vi "readMeasFromFile.vi"(0 "path":path) -> (1 "data":T1(array[cluster]), 2 "Count":i32)   [LabVIEW 2010]
panel:
  out "error out":errorcluster
  in  "MeasData":T2
  in  "Array":string[](array[string])
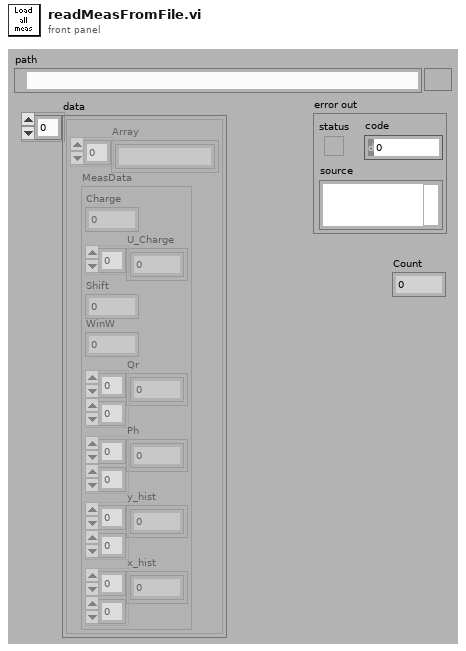
[diagram p1: front panel]
types:
  T1 = cluster{"Array":string[], "MeasData":cluster{"Charge":i32, "U_Charge":i32[], "Shift":i32, "WinW":i32, "Qr":i32[][], "Ph":i32[][], "y_hist":i32[][], "x_hist":i32[][]}}[]
  T2 = cluster{"Charge":i32, "U_Charge":i32[], "Shift":i32, "WinW":i32, "Qr":i32[][], "Ph":i32[][], "y_hist":i32[][], "x_hist":i32[][]}
  T3 = cluster{"Array":string[], "MeasData":cluster{"Charge":i32, "U_Charge":i32[], "Shift":i32, "WinW":i32, "Qr":i32[][], "Ph":i32[][], "y_hist":i32[][], "x_hist":i32[][]}}
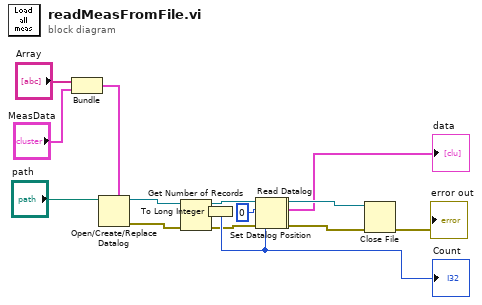
[diagram p0: block diagram]
diagram:
  n1 = Bundle("Array"="Array", "MeasData"="MeasData") -> (w9:T3)  [unwired: 1 in]
  n2 = Open/Create/Replace Datalog(5:w9, 11:"path") -> (0:w16:errorcluster, 3:w17:refnum<k1>)  [unwired: 4 in, 1 out]
  n3 = Get Number of Records(4:w16, 7:w17) -> (0:w6:errorcluster, 2:w3:i64, 3:w5:refnum<k1>)
  n4 = To Long Integer(number=w3) -> (32bit integer=w8:i32)
  "Count" <- w8
  n5 = Set Datalog Position(4:w6, 6:0, 7:w5) -> (0:w1:errorcluster, 3:w2:refnum<k1>)  [unwired: 1 in]
  n6 = Read Datalog(4:w1, 6:w8, 7:w2) -> (0:w11:errorcluster, 2:→"data":T1, 3:w12:refnum<k1>)
  n7 = Close File(refnum=w12, error in=w11) -> (error out=→"error out":errorcluster)  [unwired: 1 out]
